vi "Set Data Channel Property - ALL.vi"(8 "error in":errorcluster, 10 "Item Informations array":T2[](array[typedef]), 11 "Item Ref in":T1 format="%.0x") -> (0 "error out":errorcluster)   [LabVIEW 2023, in "Vires VTD System Explorer.lvlib"]
uses:
  Vires VTD System Explorer.lvlib
  Item Informations.ctl
  <vilib>/NI VeriStand/Custom Device API/Custom Device Item Info.ctl
  <vilib>/NI VeriStand/Custom Device API/Custom Device Channel.ctl
  <vilib>/NI VeriStand/Custom Device API/Custom Device Channel Type.ctl
  Data Channel Custom Property.ctl
  <vilib>/NI VeriStand/Custom Device API/Custom Device Item Ref.ctl
  <vilib>/NI VeriStand/Custom Device API/Custom Device API.lvlib
  <vilib>/NI VeriStand/Custom Device Tools/Custom Device Utility Library/Custom Device Utility Library.lvlib
  <vilib>/NI VeriStand/Custom Device Tools/Custom Device Utility Library/NI VeriStand - Search for Item by GUID.vi
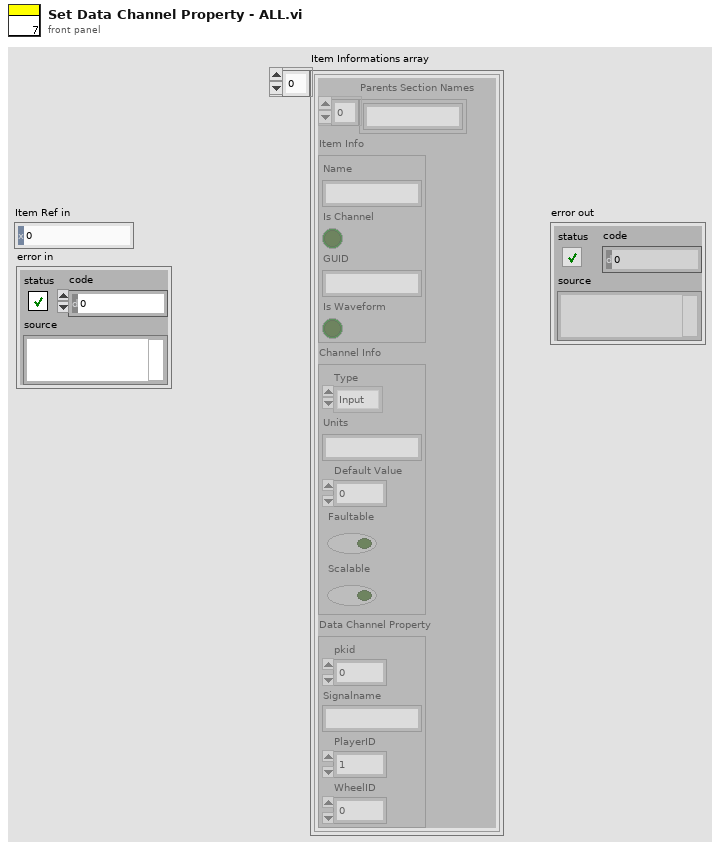
[diagram p1: front panel]
types:
  T1 = typedef "Custom Device API.lvlib/Custom Device Item Ref.ctl" = u64
  T2 = typedef "Vires VTD System Explorer.lvlib/Item Informations.ctl" = cluster{"Parents Section Names":string[], "Item Info":T3, "Channel Info":T4, "Data Channel Property":T6}
  T3 = typedef "Custom Device API.lvlib/Custom Device Item Info.ctl" = cluster{"Name":string, "Is Channel":bool, "GUID":string, "Is Waveform":bool}
  T4 = typedef "Custom Device API.lvlib/Custom Device Channel.ctl" = cluster{"Type":T5, "Units":string, "Default Value":dbl, "Faultable":bool, "Scalable":bool}
  T5 = typedef "Custom Device API.lvlib/Custom Device Channel Type.ctl" = enum16{"Input", "Output"}
  T6 = typedef "Vires VTD System Explorer.lvlib/Data Channel Custom Property.ctl" = cluster{"pkid":u32, "Signalname":string, "PlayerID":u8, "WheelID":i32}
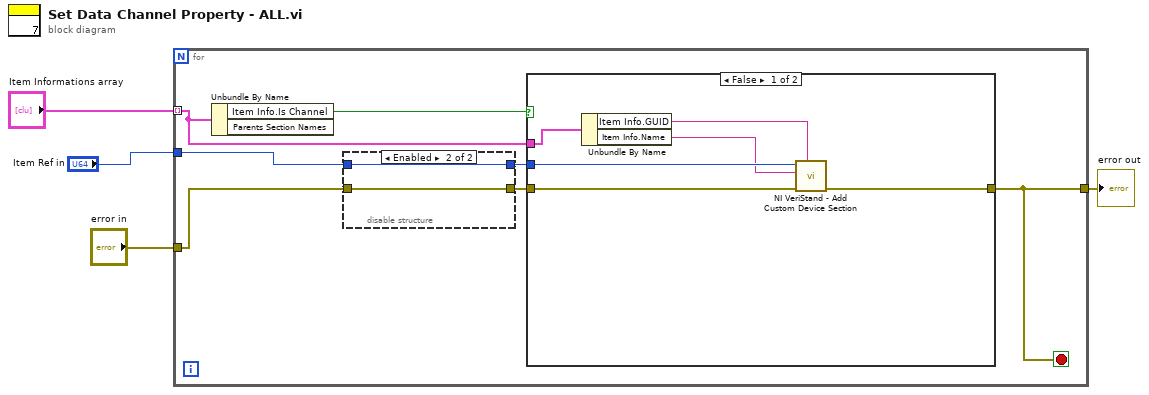
[diagram p0: block diagram]
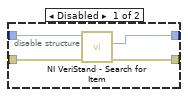
[diagram p2: hidden frame]
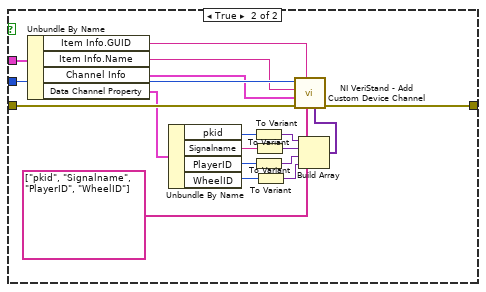
[diagram p3: hidden frame]
diagram:
  n1 = for {
    tunnel: "Item Informations array" -> [w10] mode=indexing
    tunnel: [w6] -> w1
    tunnel: "error in" -> [w7]
    tunnel: "Item Ref in" -> [w5]
    stop <- w6 stop-if-true
    n2 = Unbundle By Name(w10) -> ("Item Info.Is Channel"=w11:bool)  [unwired: 1 out]
    n3 = disable-structure shown="Enabled" {
      disable-tunnel: [w15 w17] -> w9
      disable-tunnel: [w14 w16] -> w8
      disable-tunnel: w7 -> [w13 w16]
      disable-tunnel: w5 -> [w12 w17]
      frame Disabled {
        n4 = call-poly <vilib>:"NI VeriStand - Search for Item.vi"("error in"=w13, "Section Ref in"=w12) -> ("error out"=w14:errorcluster, "Item Ref"=w15:T1)  [unwired: 6 in, 2 out]
      }
      frame Enabled {
      }
    }
    n5 = case shown="False" w11 {
      tunnel: w9 -> [w23 w41]
      tunnel: w10 -> [w22 w40]
      tunnel: w8 -> [w19 w36]
      tunnel: [w18 w35] -> w6
      frame False {
        n6 = Unbundle By Name(w22) -> ("Item Info.GUID"=w21:string, "Item Info.Name"=w20:string)
        n7 = call <vilib>:"NI VeriStand - Add Custom Device Section.vi"("GUID (Default Section)"=w21, "error in (no error)"=w19, "Section Name"=w20, "Parent Ref in"=w23) -> ("error out"=w18:errorcluster)  [unwired: 4 in, 3 out]
      }
      frame True {
        n8 = Unbundle By Name(w40) -> ("Item Info.GUID"=w38:string, "Item Info.Name"=w39:string, "Channel Info"=w37:T4, "Data Channel Property"=w34:T6)
        n9 = Unbundle By Name(w34) -> ("pkid"=w28:u32, "Signalname"=w27:string, "PlayerID"=w26:u8, "WheelID"=w25:i32)
        n10 = To Variant(anything=w28) -> (Variant=w31:variant)
        n11 = To Variant(anything=w26) -> (Variant=w30:variant)
        n12 = To Variant(anything=w27) -> (Variant=w29:variant)
        n13 = To Variant(anything=w25) -> (Variant=w32:variant)
        n14 = Build Array(w31, w29, w30, w32) -> (w24:variant[])
        n15 = call <vilib>:"NI VeriStand - Add Custom Device Channel.vi"("Property Values"=w24, "Property names"=string[] ["pkid", "Signalname", "PlayerID", "WheelID"], "GUID (Default Channel)"=w38, "error in (no error)"=w36, "Channel"=w37, "Channel Name"=w39, "Parent Ref in"=w41) -> ("error out"=w35:errorcluster)  [unwired: 1 in, 3 out]
      }
    }
  }
  "error out" <- w1
